vi "Global - RT Stream Connections.vi"() -> ()   [LabVIEW 2013]
uses:
  support/Message Queue/Message Cluster.ctl
  support/Message Queue/Message Queue.lvlib
panel:
  in  "RT Writer Stream":refnum<k21> caption="RT写入方流"
  in  "UI Writer Stream":refnum<k21> caption="UI写入方流"
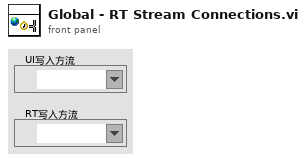
[diagram p1: front panel]
diagram:
